vi "libdaq_error.vi"(8 "error source":string, 9 "error code":i32, 11 "错误输入（无错误）":errorcluster) -> (3 "错误输出":errorcluster)   [LabVIEW 2010, in "libdaqVI.lvlib"]
uses:
  libdaqVI.lvlib
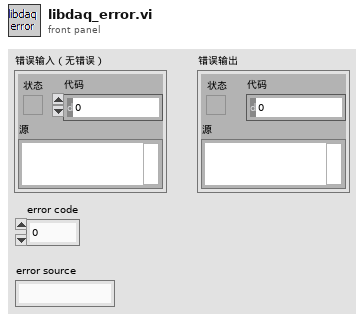
[diagram p1: front panel]
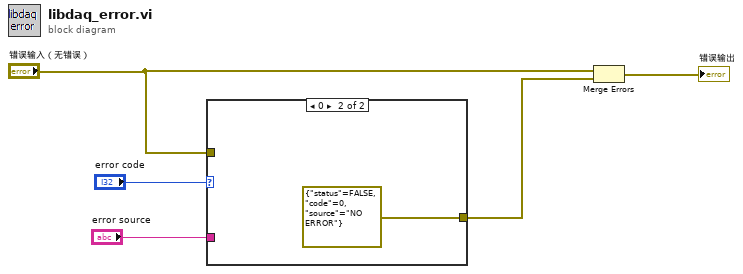
[diagram p0: block diagram]
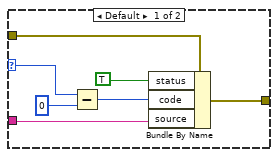
[diagram p2: hidden frame]
diagram:
  n1 = case shown="0" "error code" {
    selector: "error code" -> [w8 _]
    tunnel: [w12 errorcluster {"status"=FALSE, "code"=0, "source"="NO ERROR"} ("错误输入")] -> w4
    tunnel: "error source" -> [w10 _]
    tunnel: "错误输入（无错误）" -> [w6 _]
    frame Default {
      n2 = Subtract(x=w8, y=0) -> (x-y=w9:i32)
      n3 = Bundle By Name(cluster=w6, "status"=TRUE, "code"=w9, "source"=w10) -> (w12:errorcluster)
    }
    frame 0 {
    }
  }
  n4 = Merge Errors("错误输入（无错误）", w4) -> (→"错误输出":errorcluster)
